vi "To CSV File.vi"(8 "error in (no error)":errorcluster, 9 "Path":path, 10 "engine configuration":refnum<class "engine configuration.lvclass">, 11 "Increment editor node in":refnum<class "Increment editor node.lvclass">) -> (0 "error out":errorcluster, 3 "Increment editor node out":refnum<class "Increment editor node.lvclass">)   [LabVIEW 2015, in "Increment editor node.lvclass"]
uses:
  Increment editor node.lvclass
  <vilib>/NI/Module Execution Interface/Engine Configuration/engine configuration.lvclass
  module/configuration/Increment configuration.lvclass
  <vilib>/NI/Configuration Framework/serializable configuration/NISE_CEF_serializable configuration.lvclass/NISE_CEF_serializable configuration.ctl
  module/configuration/Increment configuration.lvclass/Increment configuration.ctl
  <vilib>/NI/Tag Bus/tag/tag descriptor.lvclass/tag descriptor.ctl
  <vilib>/Utility/LVClass/Get LV Class Name.vi
  <vilib>/NI/Configuration Framework/error generator/NISE_error generator.vi
  <vilib>/NI/Tag Bus Module Framework/channel/TBM channel.lvclass
  <vilib>/NI/Configuration Framework/serializable configuration/NISE_CEF_serializable configuration.lvclass
  <vilib>/NI/Tag Bus/tag/tag descriptor.lvclass
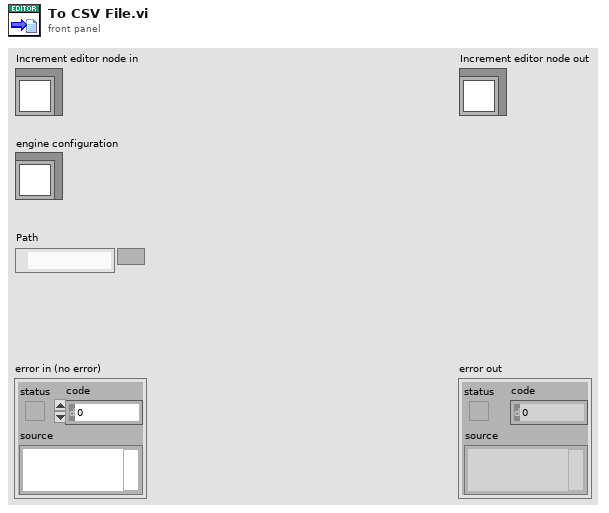
[diagram p1: front panel]
types:
  T1 = typedef "Increment configuration.lvclass/Line.ctl" = cluster{"Name":string, "channel in":refnum<class "TBM channel.lvclass">, "channel out":refnum<class "TBM channel.lvclass">}
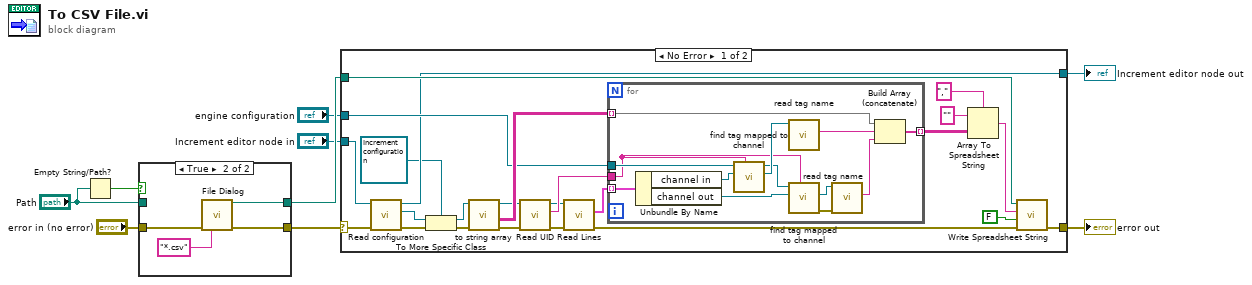
[diagram p0: block diagram]
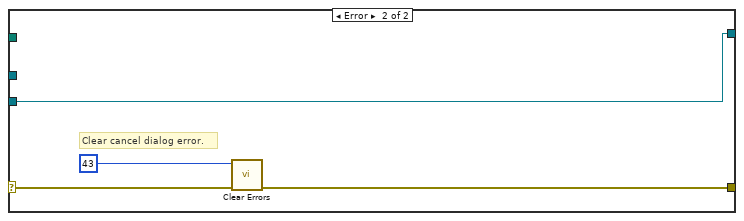
[diagram p3: hidden frame]
diagram:
  n1 = Empty String/Path?(string/path="Path") -> (empty?=w9:bool)
  n2 = case shown="True" w9 {
    tunnel: "error in (no error)" -> [w10 w14]
    tunnel: [w10 w13] -> w7
    tunnel: [w11 w12] -> w8
    tunnel: "Path" -> [w11 _]
    frame False {
    }
    frame True {
      n3 = call "File Dialog"("error in"=w14, "pattern (all files)"="*.csv") -> ("selected path"=w12:path, "error out"=w13:errorcluster)  [unwired: 10 in, 2 out]
    }
  }
  n4 = case shown="No Error" w7 {
    selector: w7 -> [w26 w55]
    tunnel: [w37 w54] -> w2
    tunnel: [w25 w56] -> w1
    tunnel: "Increment editor node in" -> [w27 w56]
    tunnel: w8 -> [w33 _]
    tunnel: "engine configuration" -> [w30 _]
    frame No Error {
      n5 = call-dynamic "Read configuration.vi"("error in"=w26, "Increment editor node in"=w27) -> ("error out"=w24:errorcluster, "configuration"=w23:refnum<class "NISE_CEF_serializable configuration.lvclass">, "Increment editor node out"=w25:refnum<class "Increment editor node.lvclass">)  [unwired: 7 in]
      n6 = To More Specific Class(target class=refnum<class "Increment configuration.lvclass"> refnum ("tag bus configurable plugin module configuration"), reference=w23, error in=w24) -> (specific class reference=w39:refnum<class "Increment configuration.lvclass">, error out=w38:errorcluster)
      n7 = call-dynamic "to string array.vi"("error in (no error)"=w38, "Increment configuration in"=w39) -> ("error out"=w21:errorcluster, "Array"=w32:string[][], "Increment configuration out"=w22:refnum<class "Increment configuration.lvclass">)  [unwired: 6 in, 1 out]
      n8 = call <vilib>:"Read UID.vi"("error in"=w21, "configuration in"=w22) -> ("error out"=w19:errorcluster, "instance id"=w29:string, "configuration out"=w16:refnum<class "Increment configuration.lvclass">)  [unwired: 7 in]
      n9 = call "Read Lines.vi"("error in (no error)"=w19, "Increment configuration in"=w16) -> ("error out"=w18:errorcluster, "Lines"=w17:T1[])  [unwired: 7 in, 1 out]
      n10 = for {
        tunnel: w32 -> [w48] mode=indexing
        tunnel: [w46] -> w31 mode=indexing
        tunnel: w17 -> [w52] mode=indexing
        tunnel: w30 -> [w50]
        tunnel: w29 -> [w42]
        n11 = Unbundle By Name(w52) -> ("channel in"=w51:refnum<class "TBM channel.lvclass">, "channel out"=w41:refnum<class "TBM channel.lvclass">)
        n12 = call <vilib>:"find tag mapped to channel.vi"("owner"=w42, "channel"=w51, "engine configuration in"=w50) -> ("tag"=w49:refnum<class "tag descriptor.lvclass">, "engine configuration out"=w43:refnum<class "engine configuration.lvclass">)  [unwired: 6 in, 1 out]
        n13 = call <vilib>:"read tag name.vi"("system tag in"=w49) -> ("name"=w47:string)  [unwired: 8 in, 2 out]
        n14 = call <vilib>:"find tag mapped to channel.vi"("owner"=w42, "channel"=w41, "engine configuration in"=w43) -> ("error out"=w45:errorcluster, "tag"=w44:refnum<class "tag descriptor.lvclass">)  [unwired: 6 in, 1 out]
        n15 = call <vilib>:"read tag name.vi"("error in"=w45, "system tag in"=w44) -> ("name"=w40:string)  [unwired: 7 in, 2 out]
        n16 = Build Array (concatenate)(w48, w47, w40) -> (w46:string[])
      }
      n17 = Array To Spreadsheet String(delimiter (Tab)=",", array=w31, 3:"" ("format string")) -> (spreadsheet string=w36:string)
      n18 = call <vilib>:"Write Spreadsheet String.vi"("error in"=w18, "append to file? (new file:F)"=FALSE, "spreadsheet string"=w36, "file path (dialog if empty)"=w33) -> ("error out"=w37:errorcluster)  [unwired: 6 in, 1 out]
    }
    frame Error {
      # "Clear cancel dialog error."
      n19 = call <vilib>:"Clear Errors.vi"("error in (no error)"=w55, "specific error code to clear (0: all)"=43) -> ("error out"=w54:errorcluster)  [unwired: 4 in, 1 out]
    }
  }
  "error out" <- w2
  "Increment editor node out" <- w1
